vi "crane_anim_loop.vi"(0 "X":dbl min=0.0 max=0.5 step=0.01, 1 "Theta":dbl step=0.1, 2 "Z":dbl step=0.01, 3 "Alpha":dbl step=0.05, 4 "Beta":dbl step=0.05, 6 "Main in":refnum<vi>(3d-picture), 7 "Target X":dbl, 9 "Target Theta":dbl, 11 "Target Z":dbl, 12 "Trolley":refnum<vi>, 14 "Arm":refnum<vi>, 15 "Load":refnum<vi>, 16 "Load Line":refnum<vi>, 17 "Pivot Alpha":refnum<vi>, 18 "Pivot Beta":refnum<vi>, 19 "Target":refnum<vi>) -> (8 "Main out":refnum<vi>(3d-picture))   [LabVIEW 2009]
uses:
  <vilib>/picture/3D Picture Control/NI_3D Picture Control.lvlib
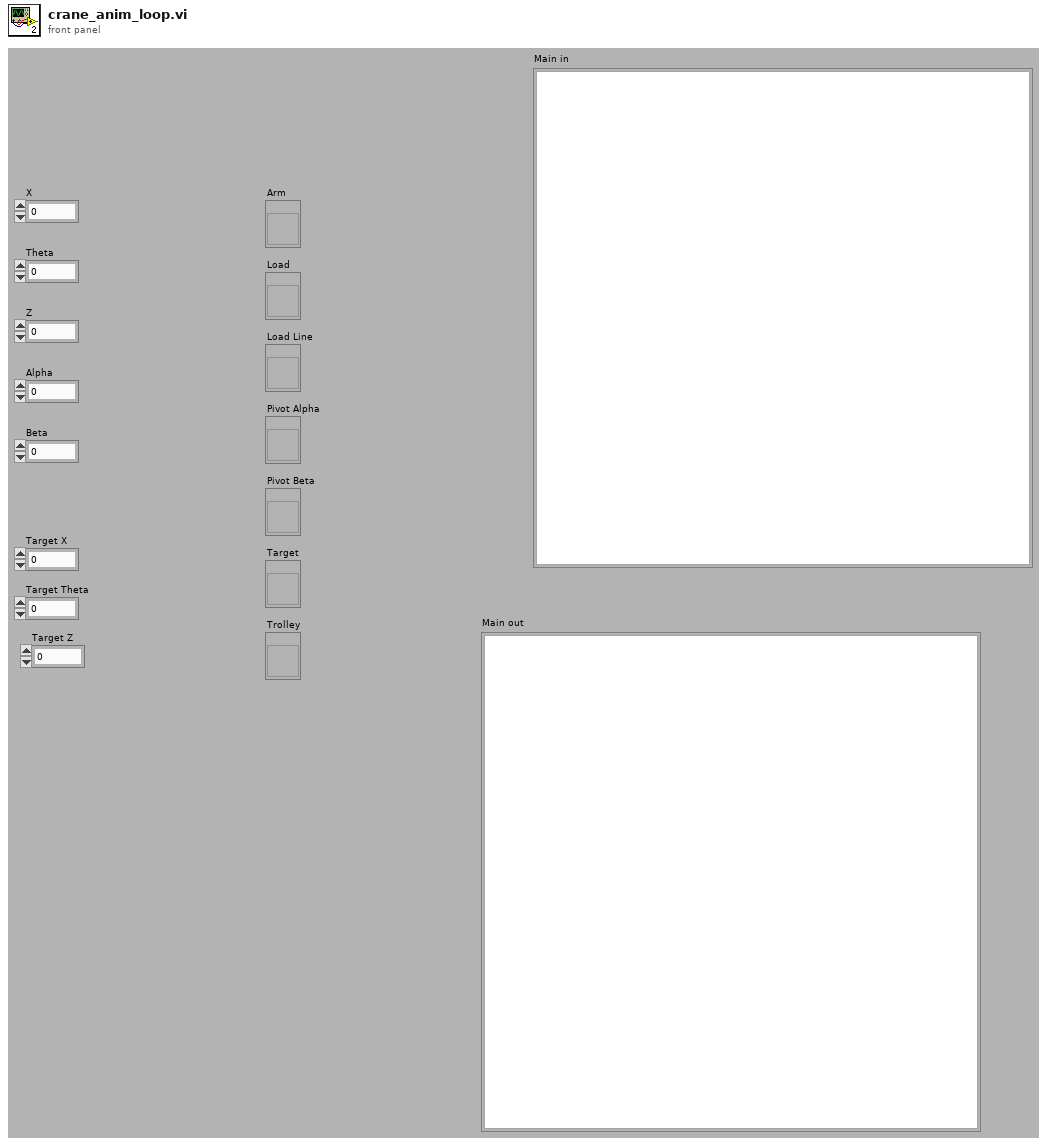
[diagram p1: front panel]
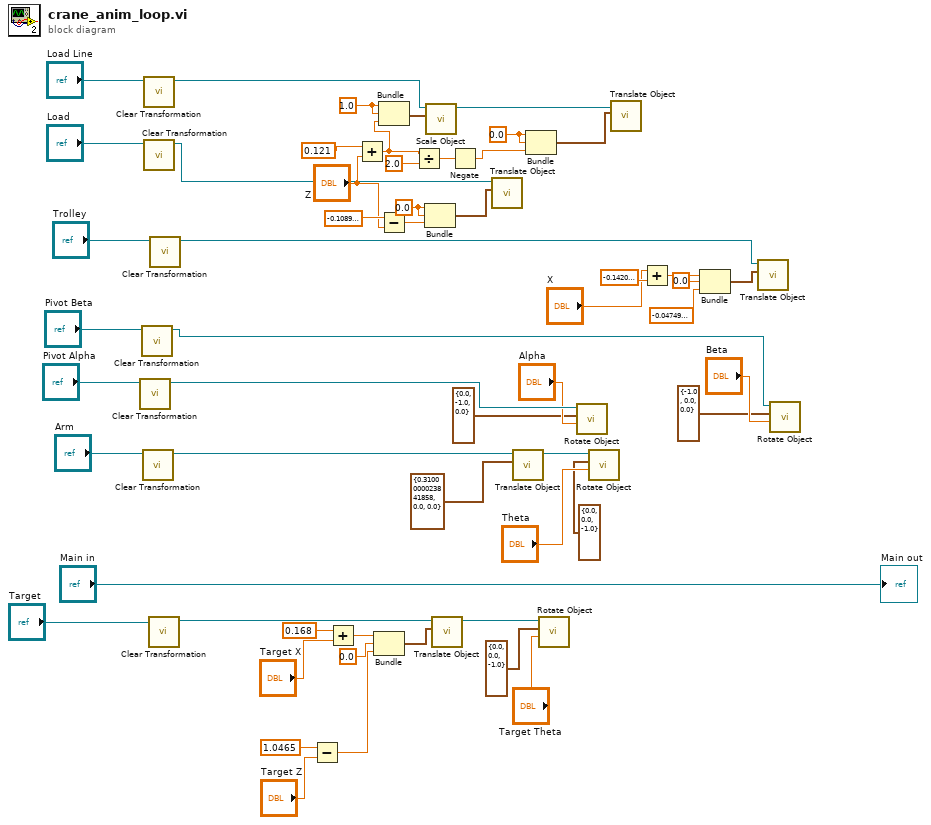
[diagram p0: block diagram]
diagram:
  w22 = sgl 0.0 ("X")
  w27 = 1.0 ("x")
  w31 = sgl 0.0 ("X")
  n1 = call <vilib>:"Clear Transformation.vi"("Object Refnum In"="Pivot Alpha") -> ("Object Refnum Out"=w53:refnum<vi>)  [unwired: 9 in, 1 out]
  n2 = call <vilib>:"Clear Transformation.vi"("Object Refnum In"="Pivot Beta") -> ("Object Refnum Out"=w52:refnum<vi>)  [unwired: 9 in, 1 out]
  n3 = call <vilib>:"Clear Transformation.vi"("Object Refnum In"="Arm") -> ("Object Refnum Out"=w54:refnum<vi>)  [unwired: 9 in, 1 out]
  n4 = call <vilib>:"Clear Transformation.vi"("Object Refnum In"="Load Line") -> ("Object Refnum Out"=w50:refnum<vi>)  [unwired: 9 in, 1 out]
  n5 = call <vilib>:"Clear Transformation.vi"("Object Refnum In"="Load") -> ("Object Refnum Out"=w55:refnum<vi>)  [unwired: 9 in, 1 out]
  n6 = call <vilib>:"Clear Transformation.vi"("Object Refnum In"="Target") -> ("Object Refnum Out"=w49:refnum<vi>)  [unwired: 9 in, 1 out]
  n7 = call <vilib>:"Clear Transformation.vi"("Object Refnum In"="Trolley") -> ("Object Refnum Out"=w51:refnum<vi>)  [unwired: 9 in, 1 out]
  n8 = Subtract(x=1.0465, y="Target Z") -> (x-y=w13:dbl)
  n9 = Add(x=0.168, y="Target X") -> (x+y=w11:dbl)
  n10 = Add(x=0.121, y="Z") -> (x+y=w25:dbl)
  n11 = Bundle(w11, "x"=0.0, w13) -> (w16:cluster{dbl, "x":dbl, dbl})  [unwired: 1 in]
  n12 = Bundle("x"=w27, "x"=w27, w25) -> (w28:cluster{"x":dbl, "x":dbl, dbl})  [unwired: 1 in]
  n13 = Subtract(x=sgl -0.109 ("Z"), y="Z") -> (x-y=w32:dbl)
  n14 = Divide(x=w25, y=2.0) -> (x/y=w20:dbl)
  n15 = Bundle("X"=w31, "X"=w31, w32) -> (w34:cluster{"X":sgl, "X":sgl, dbl})  [unwired: 1 in]
  n16 = call <vilib>:"Scale Object.vi"("Scale"=w28, "Scene.Object In"=w50) -> ("Scene.Object Out"=w26:refnum<vi>)  [unwired: 8 in, 1 out]
  n17 = call <vilib>:"Translate Object.vi"("Translation"=w16, "Scene.Object In"=w49) -> ("Scene.Object Out"=w19:refnum<vi>)  [unwired: 8 in, 1 out]
  n18 = Negate(x=w20) -> (-x=w21:dbl)
  n19 = call <vilib>:"Translate Object.vi"("Translation"=w34, "Scene.Object In"=w55) -> ()  [unwired: 8 in, 2 out]
  n20 = call <vilib>:"Translate Object.vi"("Translation"=cluster{"X":sgl, "Y":sgl, "Z":sgl} {"X"=0.31, "Y"=0.0, "Z"=0.0}, "Scene.Object In"=w54) -> ("Scene.Object Out"=w46:refnum<vi>)  [unwired: 8 in, 1 out]
  n21 = Bundle("X"=w22, "X"=w22, w21) -> (w23:cluster{"X":sgl, "X":sgl, dbl})  [unwired: 1 in]
  n22 = call <vilib>:"Rotate Object.vi"("Angle"="Target Theta", "Axis"=cluster{"X":sgl, "Y":sgl, "Z":sgl} {"X"=0.0, "Y"=0.0, "Z"=-1.0}, "Scene.Object In"=w19) -> ()  [unwired: 7 in, 2 out]
  n23 = call <vilib>:"Rotate Object.vi"("Angle"="Alpha", "Axis"=cluster{"X":sgl, "Y":sgl, "Z":sgl} {"X"=0.0, "Y"=-1.0, "Z"=0.0}, "Scene.Object In"=w53) -> ()  [unwired: 7 in, 2 out]
  n24 = call <vilib>:"Rotate Object.vi"("Angle"="Theta", "Axis"=cluster{"X":sgl, "Y":sgl, "Z":sgl} {"X"=0.0, "Y"=0.0, "Z"=-1.0}, "Scene.Object In"=w46) -> ()  [unwired: 7 in, 2 out]
  n25 = call <vilib>:"Translate Object.vi"("Translation"=w23, "Scene.Object In"=w26) -> ()  [unwired: 8 in, 2 out]
  n26 = Add(x="X", y=sgl -0.142 ("X")) -> (x+y=w39:dbl)
  n27 = Bundle(w39, "Y"=sgl 0.0, "Z"=sgl -0.0475) -> (w36:cluster{dbl, "Y":sgl, "Z":sgl})  [unwired: 1 in]
  n28 = call <vilib>:"Translate Object.vi"("Translation"=w36, "Scene.Object In"=w51) -> ()  [unwired: 8 in, 2 out]
  n29 = call <vilib>:"Rotate Object.vi"("Angle"="Beta", "Axis"=cluster{"X":sgl, "Y":sgl, "Z":sgl} {"X"=-1.0, "Y"=0.0, "Z"=0.0}, "Scene.Object In"=w52) -> ()  [unwired: 7 in, 2 out]
  "Main out" <- "Main in"
